vi "Configure Camera Attributes.vi"(6 "Exposure":i64, 7 "Gain":i64, 8 "Error In":errorcluster, 9 "Brightness":i64, 10 "Contrast":i64, 11 "Camera In":T1="cam1") -> (0 "Error Out":errorcluster, 3 "Camera Out":T1="cam1")   [LabVIEW 2018]
uses:
  <vilib>/userdefined/High Color/IMAQdx.ctl
  <resource>/objmgr/imaqdx.rc
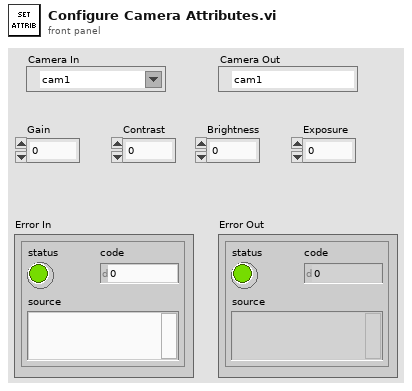
[diagram p1: front panel]
types:
  T1 = typedef "IMAQdx.ctl" = refnum<k21>
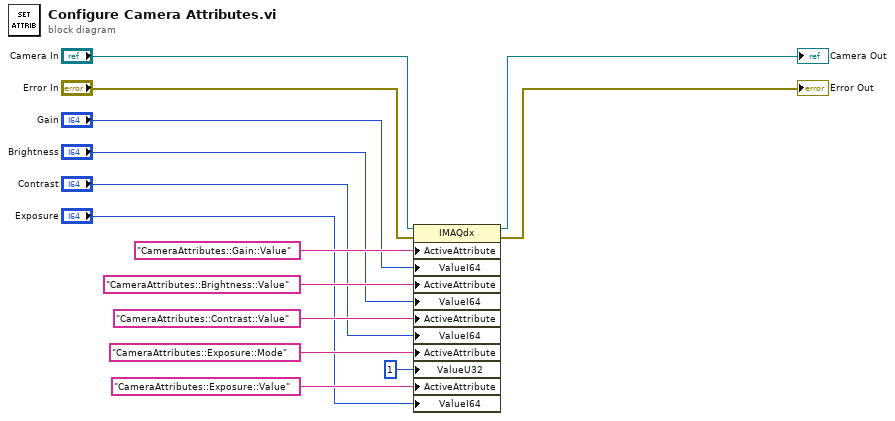
[diagram p0: block diagram]
diagram:
  n1 = property class="IMAQdx"(reference="Camera In", error in="Error In", "ActiveAttribute"="CameraAttributes::Gain::Value", "ValueI64"="Gain", "ActiveAttribute"="CameraAttributes::Brightness::Value", "ValueI64"="Brightness", "ActiveAttribute"="CameraAttributes::Contrast::Value", "ValueI64"="Contrast", "ActiveAttribute"="CameraAttributes::Exposure::Mode", "ValueU32"=u32 1, "ActiveAttribute"="CameraAttributes::Exposure::Value", "ValueI64"="Exposure") -> (reference out=→"Camera Out":T1, error out=→"Error Out":errorcluster)
